vi "target.vi"() -> ()   [LabVIEW 2020]
uses:
  <vilib>/rvi/interface/RandomDataEmulation/niFpgaRandomDataHandleErrors.vi
  <vilib>/rvi/DataTransferAndStorage/Container/XNode/niFpgaContainer.xnode
  <vilib>/rvi/interface/RandomDataEmulation/nirviRandomDataFpgaReadWriteTemplate.vi
panel:
  out "divide by zero detected":bool
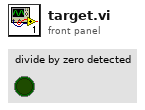
[diagram p1: front panel]
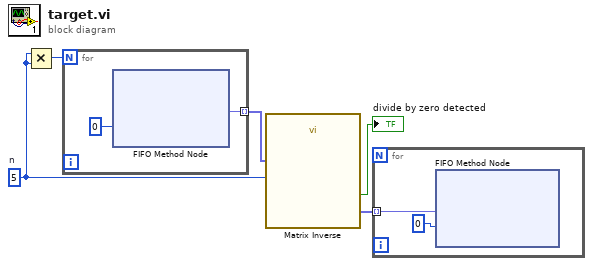
[diagram p0: block diagram]
diagram:
  w1 = 5  # n
  n1 = Multiply(x=w1, y=w1) -> (x*y=w2:i32)
  n2 = for {
    N: w2 -> [_]
    tunnel: [w7] -> w5 mode=indexing
    n3 = xnode ("FIFO Method Node")("Timeout"=0) -> ("Element"=w7:fxp<+/-,32,16>)  [unwired: 1 in, 2 out]
  }
  n4 = call "Matrix Inverse.vi"("n"=w1, "A"=w5) -> ("divide by zero detected"=→"divide by zero detected":bool, "inv(A)"=w3:fxp<+/-,32,16>[])
  n5 = for {
    tunnel: w3 -> [w9] mode=indexing
    n6 = xnode ("FIFO Method Node")("Element"=w9, "Timeout"=0) -> ()  [unwired: 1 in, 2 out]
  }
